vi "MV3D RGBD Close Device.vi"(11 "handle":u32) -> (2 "function return":i32, 3 "handle out":u32)   [LabVIEW 2015, in "Mv3dRgbd.lvlib"]
doc: "MV3D_RGBD_API MV3D_RGBD_STATUS MV3D_RGBD_CloseDevice(HANDLE *handle);"
uses:
  <userlib>/Mv3dRgbd/Mv3dRgbd.lvlib
  <userlib>/Mv3dRgbd/Mv3dRgbd.dll
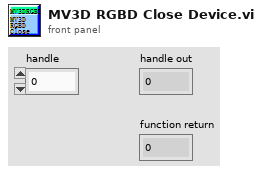
[diagram p1: front panel]
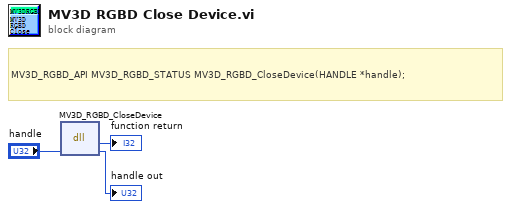
[diagram p0: block diagram]
diagram:
  # "MV3D_RGBD_API MV3D_RGBD_STATUS MV3D_RGBD_CloseDevice(HANDLE *handle);"
  n1 = dll-call lib="C:/Program Files (x86)/National Instruments/LabVIEW 2015/user.lib/Mv3dRgbd/Mv3dRgbd.*" fn="MV3D_RGBD_CloseDevice"("handle"="handle") -> (→"function return":i32, "handle"=→"handle out":u32)  [unwired: 3 in, 2 out]
